vi "Get Phasor Ratio.vi"(7 "z (NaN)":csg=nan+0.0i, 8 "Error In":errorcluster, 9 "Reference Phasor 2":T1, 10 "Reference Phasor 1":T1, 11 "Phasor":T1) -> (0 "Error Out":errorcluster, 3 "Phasor Ratio":sgl)   [LabVIEW 2019]
doc: "Computes the phasor ratio based on phasor references 1 and 2.\nIf <B>z</B> is not connected, the <B>Phasor Ratio</B> cluster is used instead."
uses:
  Phasor (g, s).ctl
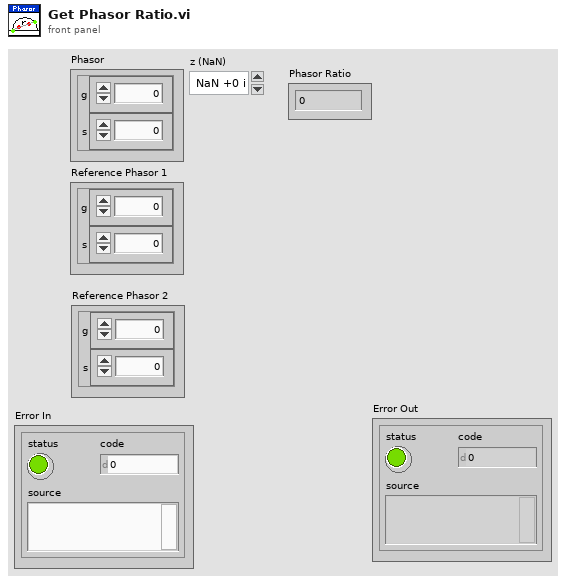
[diagram p1: front panel]
types:
  T1 = typedef "Phasor (g, s).ctl" = cluster{"g":dbl, "s":dbl}
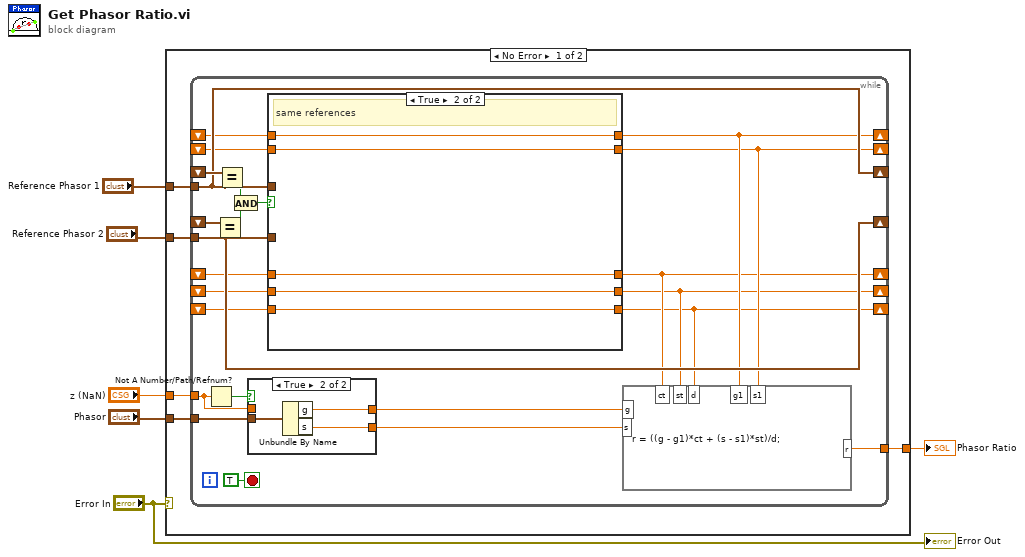
[diagram p0: block diagram]
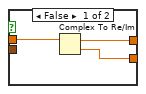
[diagram p2: hidden frame]
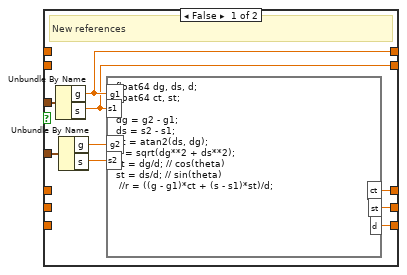
[diagram p3: hidden frame]
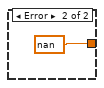
[diagram p4: hidden frame]
diagram:
  n1 = case shown="No Error" "Error In" {
    tunnel: "Reference Phasor 2" -> [w11 _]
    tunnel: "Reference Phasor 1" -> [w10 _]
    tunnel: "Phasor" -> [w9 _]
    tunnel: [w8 sgl nan ("r")] -> w3
    tunnel: "z (NaN)" -> [w7 _]
    frame No Error {
      n2 = while {
        tunnel: w11 -> [w32]
        tunnel: w10 -> [w30]
        tunnel: w9 -> [w35]
        shift-right: [w30] -> _
        shift-left: _ -> [w31]
        shift-right: [w32] -> _
        shift-left: _ -> [w33]
        shift-right: [w19] -> _
        shift-left: _ -> [w26]
        shift-right: [w18] -> _
        shift-left: _ -> [w25]
        shift-right: [w17] -> _
        shift-left: _ -> [w24]
        shift-right: [w21] -> _
        shift-left: _ -> [w23]
        shift-right: [w20] -> _
        shift-left: _ -> [w22]
        tunnel: [w14] -> w8
        tunnel: w7 -> [w12]
        stop <- TRUE stop-if-true
        n3 = Not A Number/Path/Refnum?(number/path/refnum=w12) -> (NaN/Path/Refnum?=w13:bool)
        n4 = Equal?(x=w33, y=w32) -> (x = y?=w29:bool)
        n5 = Equal?(x=w31, y=w30) -> (x = y?=w28:bool)
        n6 = And(x=w28, y=w29) -> (x .and. y?=w27:bool)
        n7 = case shown="True" w13 {
          tunnel: w35 -> [_ w41]
          tunnel: [w37 w40] -> w16
          tunnel: [w36 w39] -> w15
          tunnel: w12 -> [w38 _]
          frame False {
            n8 = Complex To Re/Im(x + iy=w38) -> (x=w37:sgl, y=w36:sgl)
          }
          frame True {
            n9 = Unbundle By Name(w41) -> ("g"=w40:dbl, "s"=w39:dbl)
          }
        }
        n10 = case shown="True" w27 {
          tunnel: w32 -> [w50 _]
          tunnel: w30 -> [w49 _]
          tunnel: [w46 w53] -> w17
          tunnel: [w45 w54] -> w18
          tunnel: [w44 w55] -> w19
          tunnel: w26 -> [_ w55]
          tunnel: w25 -> [_ w54]
          tunnel: w24 -> [_ w53]
          tunnel: [w43 w52] -> w21
          tunnel: [w42 w51] -> w20
          tunnel: w23 -> [_ w52]
          tunnel: w22 -> [_ w51]
          frame False {
            # "New references"
            n11 = Unbundle By Name(w49) -> ("g"=w43:dbl, "s"=w42:dbl)
            n12 = Unbundle By Name(w50) -> ("g"=w48:dbl, "s"=w47:dbl)
            n13 = formula code="float64 dg, ds, d;\nfloat64 ct, st;\n\ndg = g2 - g1;\nds = s2 - s1;\n//t = atan2(ds, dg);\nd = sqrt(dg**2 + ds**2);\nct = dg/d; // cos(theta)\nst = ds/d; // sin(theta)\n //r = ((g - g1)*ct + (s - s1)*st)/d;"("g1"=w43, "s1"=w42, "g2"=w48, "s2"=w47) -> ("ct"=w44:dbl, "st"=w45:dbl, "d"=w46:dbl)
          }
          frame True {
            # "same references"
          }
        }
        n14 = formula code="r = ((g - g1)*ct + (s - s1)*st)/d;"("g1"=w21, "s1"=w20, "g"=w16, "s"=w15, "ct"=w19, "st"=w18, "d"=w17) -> ("r"=w14:dbl)
      }
    }
    frame Error {
    }
  }
  "Phasor Ratio" <- w3
  "Error Out" <- "Error In"
